vi "Get All LogData from Q.vi"(8 "error in (no error)":errorcluster) -> (0 "error out":errorcluster, 1 "Events":T1[](array[typedef]), 2 "NumElements":i32, 3 "EventLogDataQRef":refnum<queue>)   [LabVIEW 2020]
doc: "Developed by Kevin Thompson\nThompson Engineering, LLC\nkevin@thompsonengineering.net"
uses:
  TD EventLogData--cluster.ctl
  GBL DataQ Ref.vi
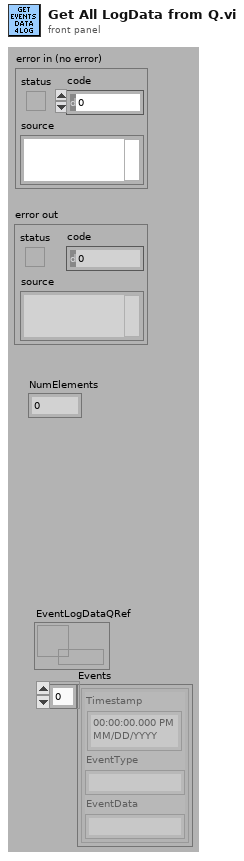
[diagram p1: front panel]
types:
  T1 = typedef "TD EventLogData--cluster.ctl" = cluster{"Timestamp":timestamp, "EventType":string, "EventData":string}
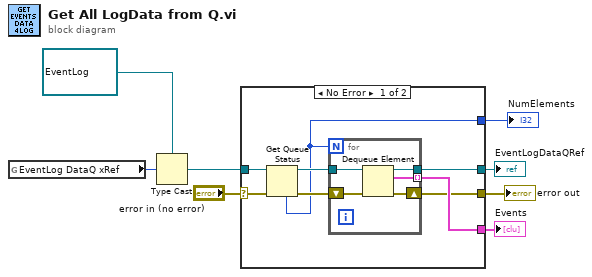
[diagram p0: block diagram]
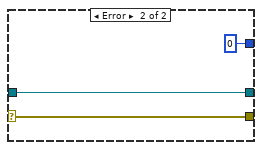
[diagram p2: hidden frame]
diagram:
  n1 = global read "GBL DataQ Ref.vi" "EventLog DataQ xRef"() -> (w4:u32)
  n2 = Type Cast(type=refnum<queue> refnum ("EventLogDataQRef"), x=w4) -> (*(type *) &x=w6:refnum<queue>)
  n3 = case shown="No Error" "error in (no error)" {
    selector: "error in (no error)" -> [w16 w23]
    tunnel: w6 -> [w15 w24]
    tunnel: [w10 w23] -> w8
    tunnel: [w14 w24] -> w2
    tunnel: [w11 _] -> w1
    tunnel: [w9 0 ("# elements in queue")] -> w5
    frame No Error {
      n4 = Get Queue Status(queue=w15, error in (no error)=w16) -> (queue out=w13:refnum<queue>, error out=w12:errorcluster, # elements in queue=w9:i32)  [unwired: 1 in, 5 out]
      n5 = for {
        N: w9 -> [_]
        tunnel: [w21] -> w11 mode=indexing
        tunnel: [w20] -> w14
        tunnel: w13 -> [w19]
        shift-right: [w18] -> w10
        shift-left: w12 -> [w17]
        n6 = Dequeue Element(queue=w19, error in (no error)=w17) -> (queue out=w20:refnum<queue>, element=w21:T1, error out=w18:errorcluster)  [unwired: 1 in, 1 out]
      }
    }
    frame Error {
    }
  }
  "error out" <- w8
  "NumElements" <- w5
  "EventLogDataQRef" <- w2
  "Events" <- w1
